vi "Check Login Status.vi"(5 "User Name":string, 7 "Password":string, 8 "error in (no error)":errorcluster, 11 "rows":string[][](array[string])) -> (0 "error out":errorcluster, 2 "Status":bool, 3 "Privilage":string)   [LabVIEW 2020]
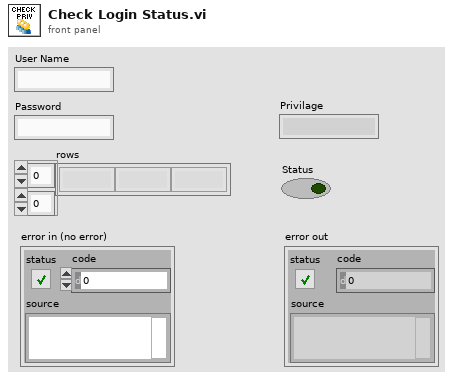
[diagram p1: front panel]
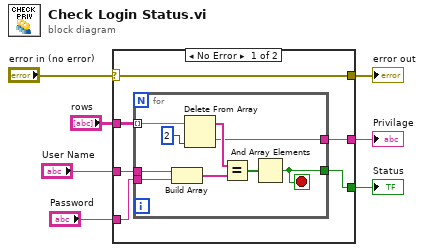
[diagram p0: block diagram]
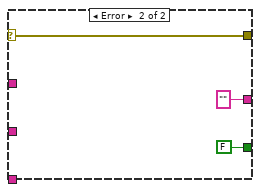
[diagram p2: hidden frame]
diagram:
  n1 = case shown="No Error" "error in (no error)" {
    selector: "error in (no error)" -> [w13 w25]
    tunnel: [w13 w25] -> w6
    tunnel: [w12 "" ("String")] -> w4
    tunnel: [w11 FALSE] -> w5
    tunnel: "rows" -> [w10 _]
    tunnel: "User Name" -> [w9 _]
    tunnel: "Password" -> [w8 _]
    frame No Error {
      n2 = for {
        tunnel: w10 -> [w22] mode=indexing
        tunnel: [w17] -> w12
        tunnel: [w16] -> w11
        tunnel: w9 -> [w15]
        tunnel: w8 -> [w14]
        stop <- w16 stop-if-true
        n3 = Build Array(w15, w14) -> (w19:string[])
        n4 = Delete From Array(array=w22, index=2) -> (deleted portion=w17:string, array with subset deleted=w20:string[])  [unwired: 1 in]
        n5 = Equal?(x=w20, y=w19) -> (x = y?=w18:bool[])
        n6 = And Array Elements(Boolean array=w18) -> (logical AND=w16:bool)
      }
    }
    frame Error {
    }
  }
  "error out" <- w6
  "Status" <- w5
  "Privilage" <- w4
